vi "initialize.vi"(0 "NInstrSim_ConfigureWaveformFormat":refnum<class "NInstrSim_ConfigureWaveformFormat.lvclass">, 3 "initializationData":variant, 5 "error in (no error)":errorcluster, 7 "binaryString":string, 8 "I8 Array":i8[](array[numeric]), 9 "prependSize? (T)":bool, 11 "byteOrder (0:big-endian, network order)":T1(ring)) -> (14 "dup NInstrSim_ConfigureWaveformFormat":refnum<class "NInstrSim_ConfigureWaveformFormat.lvclass">, 17 "found?":bool, 19 "error out":errorcluster)   [LabVIEW 2009, in "HB_Device_Examples.lvlib" / "NInstrSim_ConfigureWaveformFormat.lvclass"]
doc: "This is a dynamic dispatch VI to be implemented by child classes to initialize their attributes.\n\n<B>Recommendation:</B> Use Variant for initialization data."
uses:
  NInstrSim_ConfigureWaveformFormat.lvclass
  NInstrSim_Visitor.lvclass
  NInstrSim_ConfigureWaveformFormat.lvclass/NInstrSim_ConfigureWaveformFormat.ctl
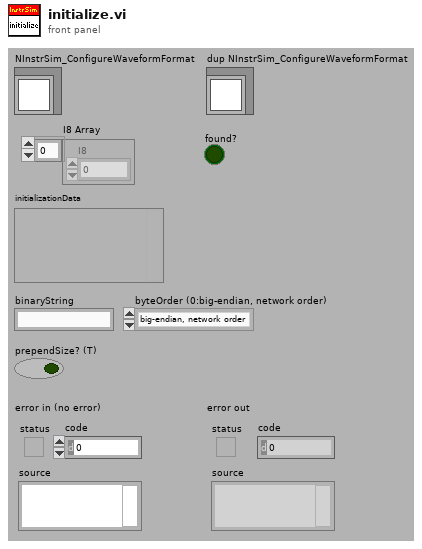
[diagram p1: front panel]
types:
  T1 = enum16{"big-endian, network order", "native, host order", "little-endian"}
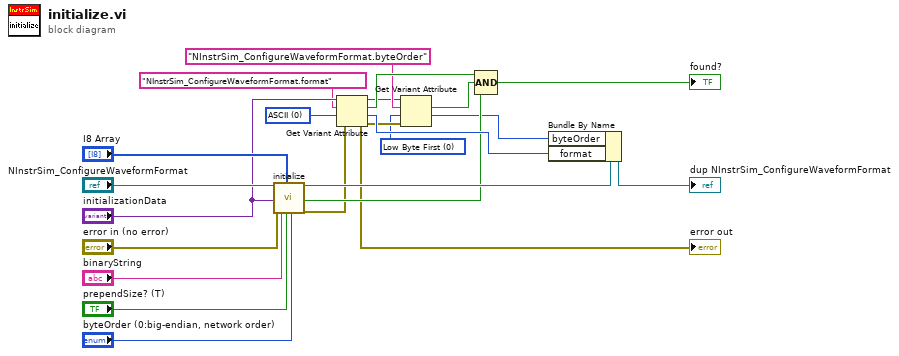
[diagram p0: block diagram]
diagram:
  w3 = u16 0 items=["Low Byte First", "High Byte First"] ("Byte Order (0:Low Byte First)")
  w7 = u16 0 items=["ASCII", "8-bit Unsigned Binary", "16-bit Signed Binary"] ("Waveform Format (0:ASCII)")
  n1 = call-parent "initialize.vi"("HGF_NetworkData"="NInstrSim_ConfigureWaveformFormat", "initializationData"="initializationData", "error in (no error)"="error in (no error)", "binaryString"="binaryString", "I8 Array"="I8 Array", "prependSize? (T)"="prependSize? (T)", "byteOrder (0:big-endian, network order)"="byteOrder (0:big-endian, network order)") -> ("dup HGF_NetworkData"=w15:refnum<class "NInstrSim_ConfigureWaveformFormat.lvclass">, "found?"=w11:bool, "error out"=w9:errorcluster)  [unwired: 10 out]
  n2 = Get Variant Attribute(Variant="initializationData", name="NInstrSim_ConfigureWaveformFormat.format", default value (empty Variant)=w7, error in=w9) -> (duplicate Variant=w5:variant, found=w12:bool, value=w13:u16, error out=w4:errorcluster)
  "error out" <- w4
  n3 = Get Variant Attribute(Variant=w5, name="NInstrSim_ConfigureWaveformFormat.byteOrder", default value (empty Variant)=w3, error in=w4) -> (found=w2:bool, value=w1:u16)  [unwired: 2 out]
  n4 = Compound Arithmetic op=AND(w12, w2, w11) -> (→"found?":bool)
  n5 = Bundle By Name(cluster=w15, "byteOrder"=w1, "format"=w13) -> (→"dup NInstrSim_ConfigureWaveformFormat":refnum<class "NInstrSim_ConfigureWaveformFormat.lvclass">)
